vi "Make Palettes for Library.vi"() -> ()   [LabVIEW 2018, in "Palette Generation.lvlib"]
uses:
  Palette Generation.lvlib
  <vilib>/Palette API/Palette Menu/Public Type Define/Palette type.ctl
  <vilib>/Palette API/Palette Menu/Palette Menu.lvlib
panel:
  in  "All files Libraries in Directory":bool
  in  "Build Class Hierarchy":bool
  in  "Done":bool
  in  "Process":bool
  out "Progress":u8(slide) scale=0.0..100.0
  in  "Overwrite Always":bool
  in  "Library Path":path
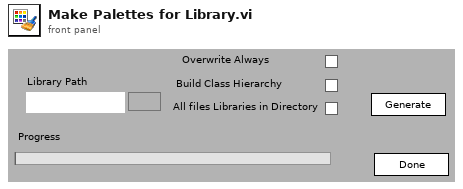
[diagram p1: front panel]
types:
  T1 = enum32{"existing file", "new file", "new or existing file", "existing dir", "new dir", "new or existing dir", "existing file (use LLBs)", "new file (use LLBs)", "new or existing file (use LLBs)", "new or existing file or directory (use LLBs)", "existing dir (use LLBs)", "new dir (use LLBs)", "new or existing dir (use LLBs)", "existing file or dir", "new file or dir", "new or existing file or dir", "existing file or dir (use LLBs)", "new file or dir (use LLBs)"}
  T2 = typedef "Palette Generation.lvlib/Palette Fiole List.ctl" = cluster{"Name":string, "Entries":cluster{string, refnum<vi>}[], "Short Name":string}
  T3 = typedef "Palette Menu.lvlib/Palette type.ctl" = i32
  T4 = typedef "Palette Menu.lvlib/Palette Data.ctl" = cluster{"display name":string, "view format":T5, "palette width":i16, "items":T6, "256 color icon":picture, "B&W color icon":picture, "help information":T8, "palette description":string, "synchronize information":T9}
  T5 = typedef "Palette Menu.lvlib/View Format.ctl" = u16
  T6 = typedef "Palette Menu.lvlib/Items.ctl" = T7[]
  T7 = typedef "Palette Menu.lvlib/Item.ctl" = cluster{"item path":path, "library path (.lvlib)":path, "use default lvlib palette":bool, "short name":string, "place VI contents":bool, "hide synchronized item":bool, "reserve spot for synch item":bool, "configure when placing VI contents":bool}
  T8 = typedef "Palette Menu.lvlib/Help Info.ctl" = cluster{"help tag":string, "help file path ":path}
  T9 = typedef "Palette Menu.lvlib/Synchronize Info.ctl" = cluster{"synchronize with directory":bool, "synchronize directory path":path}
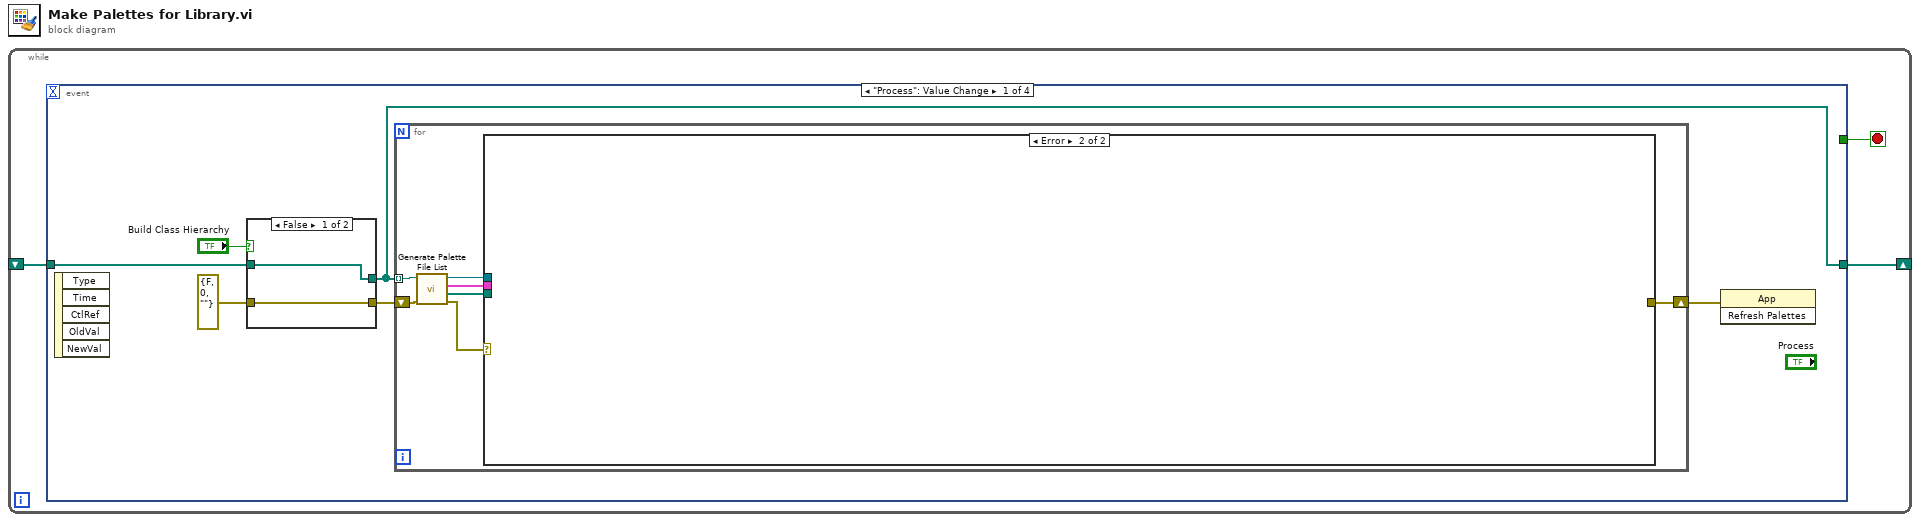
[diagram p0: block diagram]
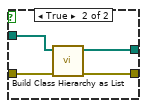
[diagram p2: hidden frame]
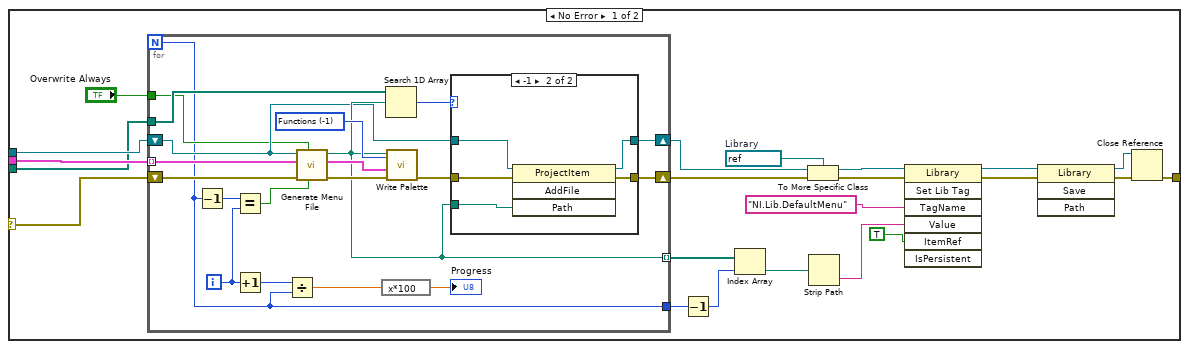
[diagram p3: hidden frame]
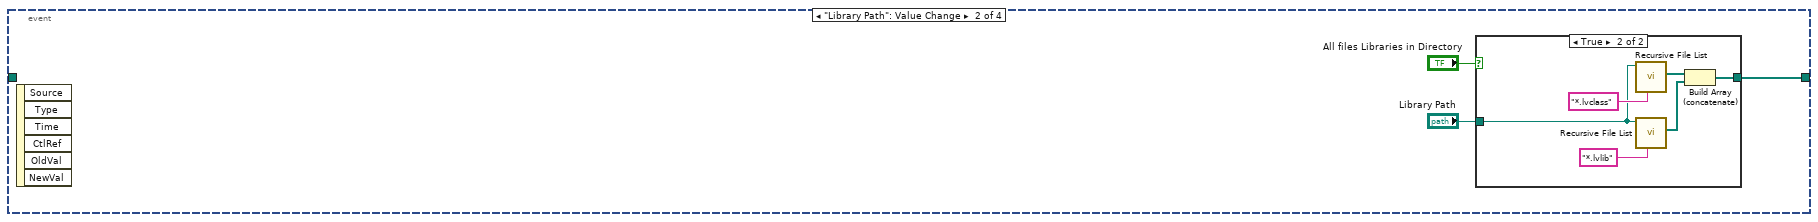
[diagram p5: hidden frame]
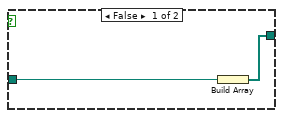
[diagram p6: hidden frame]
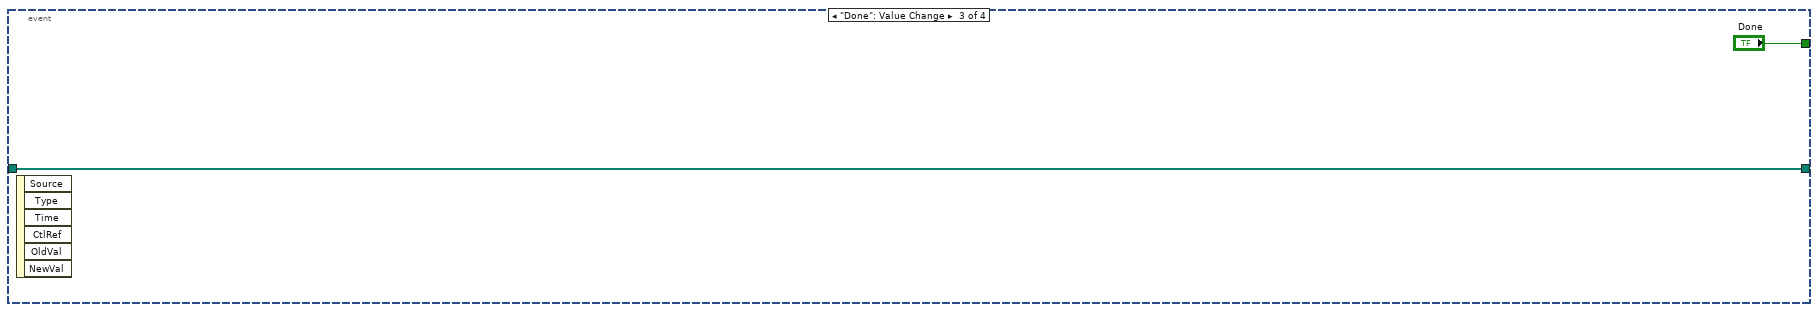
[diagram p7: hidden frame]
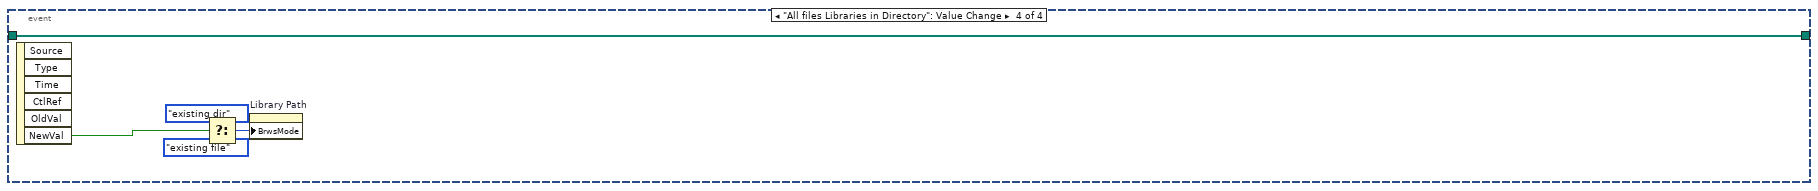
[diagram p8: hidden frame]
diagram:
  n1 = while {
    shift-right: [w2] -> _
    shift-left: _ -> [w1]
    stop <- w3 stop-if-true
    n2 = event shown="[0] \"Process\": Value Change" {
      selector: _ -> [_ _ _ _]
      dyn-events: _ -> [_ _ _ _]
      timeout: _ -> [_ _ _ _]
      tunnel: [_ _ "Done" _] -> w3
      tunnel: [w8 w73 w83 w89] -> w2
      tunnel: w1 -> [w9 _ w83 w89]
      event "Process": Value Change {
        n3 = event-data() -> ()  [unwired: 6 out]
        n4 = case shown="False" "Build Class Hierarchy" {
          tunnel: w9 -> [w11 w15]
          tunnel: [w11 w14] -> w8
          tunnel: [w10 w13] -> w5
          tunnel: errorcluster {"status"=FALSE, "code"=0, "source"=""} ("error in (no error)") -> [w10 w12]
          frame False {
          }
          frame True {
            n5 = call "Build Class Hierarchy as List.vi"("error in (no error)"=w12, "List of Class Paths"=w15) -> ("error out"=w13:errorcluster, "List of Class Paths Out"=w14:path[])  [unwired: 8 out]
          }
        }
        n6 = for {
          tunnel: w8 -> [w19] mode=indexing
          shift-right: [w17] -> w6
          shift-left: w5 -> [w18]
          n7 = call "Generate Palette File List.vi"("error in (no error)"=w18, "Library Path"=w19) -> ("error out"=w16:errorcluster, "Paths"=w20:path[], "List of Palette Files"=w22:T2[], "Library as Project item"=w21:refnum<vi>)  [unwired: 6 out]
          n8 = case shown="Error" w16 {
            selector: w16 -> [w23 _]
            tunnel: w22 -> [w44 _]
            tunnel: w21 -> [w43 _]
            tunnel: w20 -> [w39 _]
            tunnel: [w37 _] -> w17
            frame No Error {
              w40 = refnum<vi> refnum  # Library
              n9 = for {
                N -> [w45]
                tunnel: w44 -> [w64] mode=indexing
                shift-right: [w59] -> w41
                shift-left: w23 -> [w63]
                shift-right: [w58] -> w42
                shift-left: w43 -> [w54]
                tunnel: [w56] -> w33 mode=indexing
                tunnel: w39 -> [w57]
                tunnel: "Overwrite Always" -> [w52]
                tunnel: [w45] -> w31
                i -> [w48]
                w60 = T3 -1 items=["Functions"=-1, "Controls"=-2] ("palette type")
                n10 = Decrement(x=w45) -> (x-1=w49:i32)
                n11 = Equal?(x=w49, y=w48) -> (x = y?=w47:bool)
                n12 = Increment(x=w48) -> (x+1=w46:i32)
                n13 = Divide(x=w46, y=w45) -> (x/y=w51:dbl)
                n14 = call "Generate Menu File.vi"("Include Ancestor Palette ?"=w47, "Overwrite Always"=w52, "error in (no error)"=w63, "Palette Fiole List"=w64, "Library as Project item"=w54) -> ("error out"=w62:errorcluster, "palette data"=w61:T4, "Palette file path"=w56:path)  [unwired: 4 out]
                n15 = expression code="x*100"(w51) -> (→"Progress":dbl)
                n16 = Search 1D Array(1D array=w57, element=w56) -> (index of element=w55:i32)  [unwired: 1 out]
                n17 = call <vilib>:"Write Palette.vi"("error in (no error)"=w62, "palette data"=w61, "palette type"=w60, "palette path"=w56) -> ("error out"=w53:errorcluster)  [unwired: 1 in, 6 out]
                n18 = case shown="-1" w55 {
                  tunnel: [w65 w71] -> w59
                  tunnel: [w66 w70] -> w58
                  tunnel: w56 -> [_ w69]
                  tunnel: w54 -> [w66 w68]
                  tunnel: w53 -> [w65 w67]
                  frame 0, Default {
                  }
                  frame -1 {
                    n19 = invoke class="ProjectItem" method="AddFile"(reference=w68, error in=w67, "Path"=w69) -> (reference out=w70:refnum<vi>, error out=w71:errorcluster)  [unwired: 1 in, 2 out]
                  }
                }
              }
              n20 = Decrement(x=w31) -> (x-1=w30:i32)
              n21 = Index Array(array=w33, index=w30) -> (element=w32:path)
              n22 = To More Specific Class(target class=w40, reference=w42, error in=w41) -> (specific class reference=w29:refnum<vi>, error out=w26:errorcluster)
              n23 = Strip Path(path=w32) -> (name=w35:string)  [unwired: 1 out]
              n24 = invoke class="Library" method="Set Lib Tag"(reference=w29, error in=w26, "TagName"="NI.Lib.DefaultMenu" ("Tag Name"), "Value"=w35, "ItemRef"=TRUE ("Is Persistent")) -> (reference out=w28:refnum<vi>, error out=w25:errorcluster)  [unwired: 2 in, 5 out]
              n25 = invoke class="Library" method="Save"(reference=w28, error in=w25) -> (reference out=w27:refnum<vi>, error out=w24:errorcluster)  [unwired: 2 in, 2 out]
              n26 = Close Reference(reference=w27, error in (no error)=w24) -> (error out=w37:errorcluster)
            }
            frame Error {
            }
          }
        }
        n27 = invoke class="App" method="Refresh Palettes"(error in=w6) -> ()  [unwired: 2 in, 3 out]
      }
      event "Library Path": Value Change {
        n28 = event-data() -> ()  [unwired: 7 out]
        n29 = case shown="True" "All files Libraries in Directory" {
          tunnel: "Library Path" -> [w76 w81]
          tunnel: [w75 w77] -> w73
          frame False {
            n30 = Build Array(w76) -> (w75:path[])
          }
          frame True {
            n31 = call <vilib>:"Recursive File List.vi"("pattern"="*.lvclass", "Folder Path"=w81) -> ("All Files in Dir"=w79:path[])  [unwired: 2 in, 7 out]
            n32 = call <vilib>:"Recursive File List.vi"("pattern"="*.lvlib", "Folder Path"=w81) -> ("All Files in Dir"=w78:path[])  [unwired: 2 in, 7 out]
            n33 = Build Array (concatenate)(w79, w78) -> (w77:path[])
          }
        }
      }
      event "Done": Value Change {
        n34 = event-data() -> ()  [unwired: 7 out]
      }
      event "All files Libraries in Directory": Value Change {
        n35 = event-data() -> ("NewVal"=w85:bool)  [unwired: 6 out]
        n36 = Select(t=T1."existing dir" ("Browse Options:Selection Mode"), s=w85, f=T1."existing file" ("Browse Options:Selection Mode")) -> (s? t:f=w86:T1)
        n37 = property on="Library Path" class="Path"("BrwsMode"=w86) -> ()  [unwired: 2 in, 2 out]
      }
    }
  }
